vi "Search_ROI.vi"(11 "AVI File Path":path) -> (2 "ROI File Exists":bool, 3 "ROI Path":path)   [LabVIEW 2020]
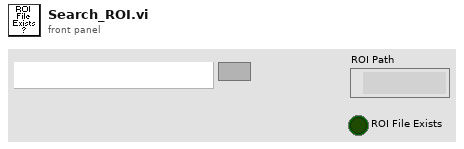
[diagram p1: front panel]
types:
  T1 = typedef "Fixed strings.ctl" = cluster{"ROI file name":string, "Normalised ROI file name":string, "Zplane Pockels values file name":string, "Functional data folder name":string, "Experiment Header file name":string, "Z-stack images folder name":string, "Groups setup rel. path":string, "Groups text file rel. path":string, "TDMS files folder name (F.img)":string, "TDMS files folder name (V.acq)":string, "TDMS files folder name (Pl.acq)":string, "Cycle rel times sequence file":string, "Dynamically called VIs folder name":string, "Time Series folder base name":string}
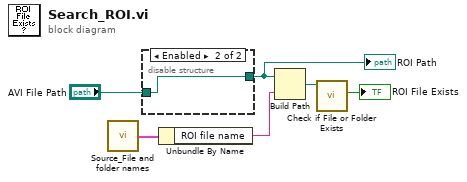
[diagram p0: block diagram]
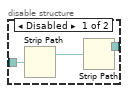
[diagram p2: hidden frame]
diagram:
  n1 = call "Source_File and folder names.vi"() -> ("Fixed strings"=w5:T1)  [unwired: 1 in]
  n2 = disable-structure shown="Enabled" {
    disable-tunnel: "AVI File Path" -> [w9 w10]
    disable-tunnel: [w7 w10] -> w1
    frame Disabled {
      n3 = Strip Path(path=w9) -> (stripped path=w8:path)  [unwired: 1 out]
      n4 = Strip Path(path=w8) -> (stripped path=w7:path)  [unwired: 1 out]
    }
    frame Enabled {
    }
  }
  "ROI Path" <- w1
  n5 = Unbundle By Name(w5) -> ("ROI file name"=w4:string)
  n6 = Build Path(base path=w1, name or relative path=w4) -> (appended path=w2:path)
  n7 = call <vilib>:"Check if File or Folder Exists.vi"("path"=w2) -> ("file or folder exists?"=→"ROI File Exists":bool)  [unwired: 8 in, 2 out]
